vi "Lookup Group.vi"(7 "Group Type (Abstract)":refnum<class "Group.lvclass">, 8 "error in (no error)":errorcluster, 10 "Group Name":string, 11 "VolatusAPI in":refnum<class "VolatusAPI.lvclass">) -> (0 "error out":errorcluster, 2 "Group":refnum<class "Group.lvclass">, 3 "VolatusAPI out":refnum<class "VolatusAPI.lvclass">)   [LabVIEW 2020, in "Volatus.lvlib" / "VolatusAPI.lvclass"]
uses:
  VolatusAPI.lvclass
  lv-vecto/Vecto/Group/Group.lvclass
  VolatusAPI.lvclass/VolatusAPI.ctl
  lv-vecto/Vecto/ChannelService/ChannelService.lvclass
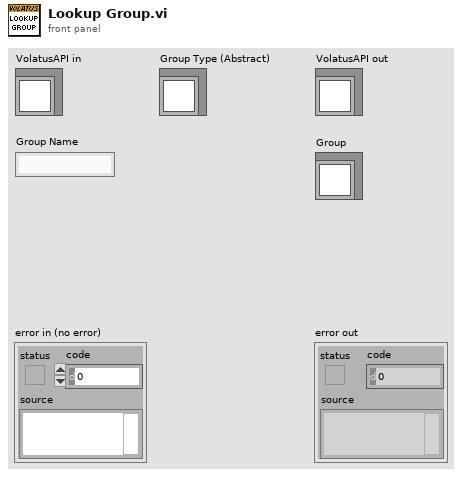
[diagram p1: front panel]
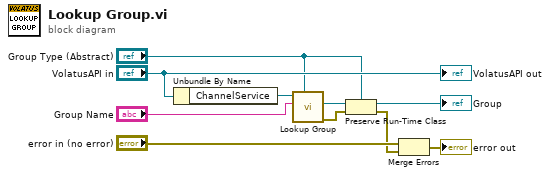
[diagram p0: block diagram]
diagram:
  n1 = Unbundle By Name("VolatusAPI in") -> ("ChannelService"=w8:refnum<class "ChannelService.lvclass">)
  n2 = call "Lookup Group.vi"("Group Type (Abstract)"="Group Type (Abstract)", "Group Name"="Group Name", "ChannelService in"=w8) -> ("error out"=w4:errorcluster, "Group"=w6:refnum<class "Group.lvclass">)  [unwired: 6 in, 1 out]
  n3 = Preserve Run-Time Class(object in=w6, error in=w4, 2:"Group Type (Abstract)") -> (object out=→"Group":refnum<class "Group.lvclass">, error out=w1:errorcluster)
  n4 = Merge Errors("error in (no error)", w1) -> (→"error out":errorcluster)
  "VolatusAPI out" <- "VolatusAPI in"
